vi "Write configuration.vi"(8 "error in (no error)":errorcluster, 11 "DAQCascade512 in":refnum<class "DAQCascade512.lvclass">) -> (0 "error out":errorcluster, 3 "DAQCascade512 out":refnum<class "DAQCascade512.lvclass">)   [LabVIEW 2012, in "DAQCascade512.lvclass"]
doc: "Writes the configuration cluster into the configuration file. Configuration file is XML-based. It's name is <component ID>.xml"
uses:
  DAQCascade512.lvclass
  <vilib>/Distrio/Murmex/Murmex/Murmex.lvclass
  DAQCascade512.lvclass/DAQCascade512.ctl
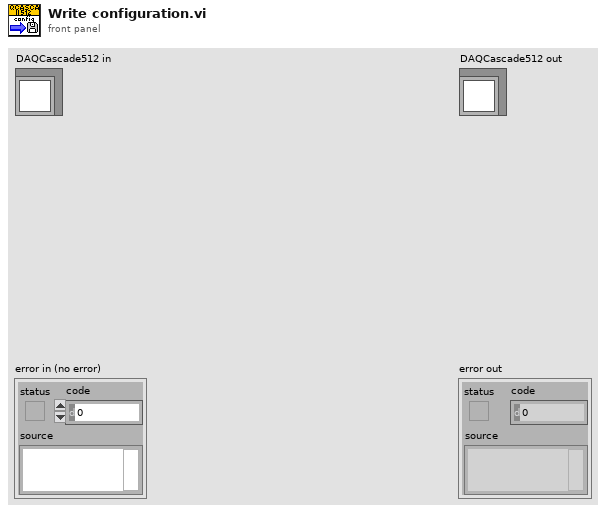
[diagram p1: front panel]
types:
  T1 = typedef "DAQCascade512.lvclass/configuration cluster.ctl" = cluster{"Camera configuration":cluster{"Temperature":dbl, "EMGain":dbl, "ClearMode":T2, "ReadoutMode":T3, "ADC Gain":T4}, "Acqusition Info":cluster{"Image type":T5, "Acquire / Focus Flag":u32}}
  T2 = typedef "Clearing_mode.ctl" = dbl
  T3 = typedef "Readout_mode.ctl" = dbl
  T4 = typedef "ADC_gain.ctl" = i32
  T5 = typedef "Image_type.ctl" = u32
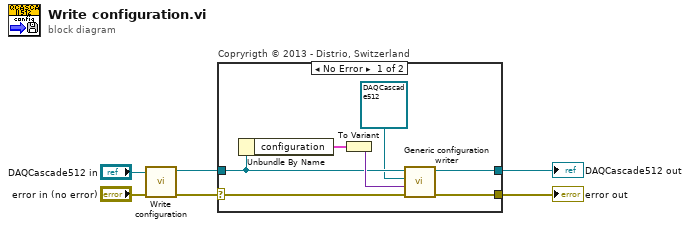
[diagram p0: block diagram]
diagram:
  n1 = call-parent "Write configuration.vi"("error in (no error)"="error in (no error)", "Murmex in"="DAQCascade512 in") -> ("error out"=w1:errorcluster, "Murmex out"=w2:refnum<class "DAQCascade512.lvclass">)  [unwired: 8 in]
  n2 = case "Copryrigth © 2013 - Distrio, Switzerland" shown="No Error" w1 {
    selector: w1 -> [w12 w15]
    tunnel: [w11 w15] -> w3
    tunnel: [w8 w14] -> w4
    tunnel: w2 -> [w9 w14]
    frame No Error {
      n3 = Unbundle By Name(w9) -> ("configuration"=w13:T1)
      n4 = To Variant(anything=w13) -> (Variant=w10:variant)
      n5 = call <vilib>:"Generic configuration writer.vi"("error in (no error)"=w12, "configuration"=w10, "inheritance level"=refnum<class "DAQCascade512.lvclass"> refnum ("DAQCascade512"), "MurmexBase in"=w9) -> ("error out"=w11:errorcluster, "MurmexBase out"=w8:refnum<class "DAQCascade512.lvclass">)  [unwired: 6 in]
    }
    frame Error {
    }
  }
  "error out" <- w3
  "DAQCascade512 out" <- w4
